vi "Clear Error if Caller is Top Level.vi"(8 "error in":errorcluster) -> (0 "error out":errorcluster, 2 "top level":bool)   [LabVIEW 2018, in "NI_TDMS File Viewer.lvlib"]
uses:
  NI_TDMS File Viewer.lvlib
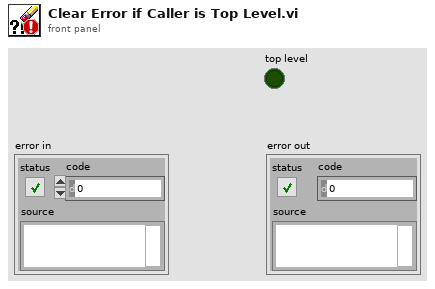
[diagram p1: front panel]
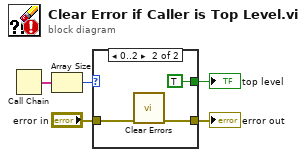
[diagram p0: block diagram]
diagram:
  n1 = Call Chain() -> (call chain=w3:string[])
  n2 = Array Size(array=w3) -> (size(s)=w2:i32)
  n3 = case shown="0..2" w2 {
    tunnel: "error in" -> [w6 w9]
    tunnel: [w6 w8] -> w4
    tunnel: [_ TRUE] -> w1
    frame Default {
      # "caller is a subVI"
    }
    frame 0..2 {
      n4 = call <vilib>:"Clear Errors.vi"("error in (no error)"=w9) -> ("error out"=w8:errorcluster)  [unwired: 5 in, 1 out]
    }
  }
  "error out" <- w4
  "top level" <- w1
